vi "Spectrograph_getEvent_rejectedCommand.vi"(8 "error in (no error)":errorcluster, 11 "logevent_rejectedCommand_Ctl":T1) -> (0 "error out":errorcluster, 2 "function return":i32, 3 "logevent_rejectedCommand_Ctl out":T1)   [LabVIEW 2016, in "SALLV_Spectrograph.lvlib"]
doc: "int Spectrograph_shm_getEvent_rejectedCommandLV(Spectrograph_logevent_rejectedCommandLV *logevent_rejectedCommand_Ctl );"
uses:
  SALLV_Spectrograph.lvlib
  DataTypes/logevent_rejectedCommand.ctl
  SALLV_Spectrograph.so
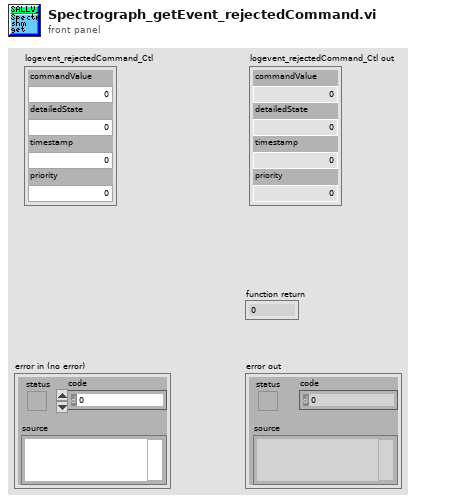
[diagram p1: front panel]
types:
  T1 = typedef "SALLV_Spectrograph.lvlib/logevent_rejectedCommand.ctl" = cluster{"commandValue":u16, "detailedState":u16, "timestamp":dbl, "priority":i32}
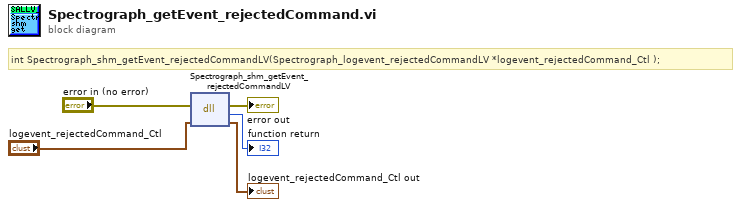
[diagram p0: block diagram]
diagram:
  # "int Spectrograph_shm_getEvent_rejectedCommandLV(Spectrograph_logevent_rejectedCommandLV *logevent_rejectedCommand_Ctl );"
  n1 = dll-call lib="home/harini/TCS/SALLV_Spectrograph/SALLV_Spectrograph.*" fn="Spectrograph_shm_getEvent_rejectedCommandLV"(error in="error in (no error)", "logevent_rejectedCommand_Ctl"="logevent_rejectedCommand_Ctl") -> (error out=→"error out":errorcluster, →"function return":i32, "logevent_rejectedCommand_Ctl"=→"logevent_rejectedCommand_Ctl out":T1)  [unwired: 2 in, 1 out]
